vi "Get Data.vi"(8 "error in (no error)":errorcluster, 11 "DAQmx Recorder in":refnum<class "DAQmx Recorder.lvclass">) -> (0 "error out":errorcluster, 2 "Data Result":refnum<class "Acquired Result.lvclass">, 3 "DAQmx Recorder out":refnum<class "DAQmx Recorder.lvclass">)   [LabVIEW 2015, in "DAQmx Recorder.lvclass"]
uses:
  DAQmx Recorder.lvclass
  NHMFL_Core/Libraries/NI-DAQ/DAQmx Digitizer/DAQmx Digitizer.lvclass
  Measure_core/Results/Acquired Result/Acquired Result.lvclass
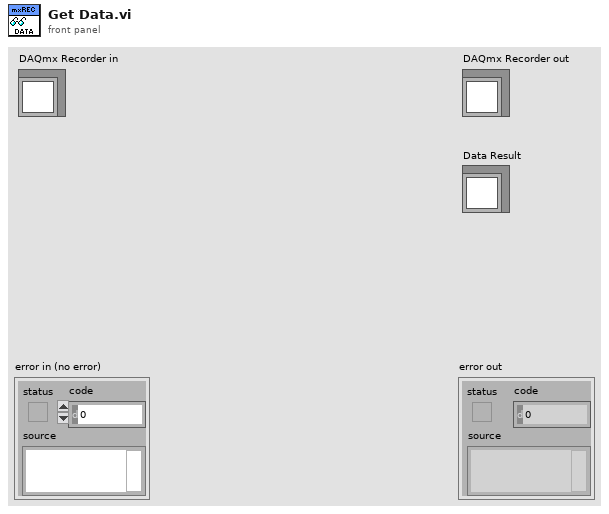
[diagram p1: front panel]
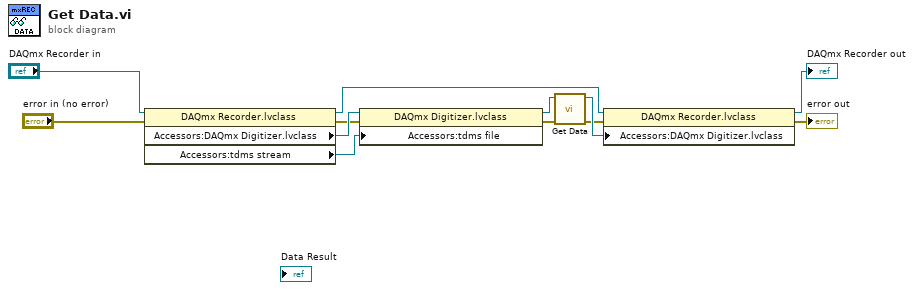
[diagram p0: block diagram]
diagram:
  n1 = property class="DAQmx Recorder.lvclass"(reference="DAQmx Recorder in", error in="error in (no error)") -> (reference out=w5:refnum<class "DAQmx Recorder.lvclass">, error out=w9:errorcluster, "Accessors:DAQmx Digitizer.lvclass"=w10:refnum<class "DAQmx Digitizer.lvclass">, "Accessors:tdms stream"=w11:refnum<k34>)
  n2 = property class="DAQmx Digitizer.lvclass"(reference=w10, error in=w9, "Accessors:tdms file"=w11) -> (reference out=w7:refnum<class "DAQmx Digitizer.lvclass">, error out=w6:errorcluster)
  n3 = call-dynamic "Get Data.vi"("error in (no error)"=w6, "DAQmx Digitizer in"=w7) -> ("error out"=w3:errorcluster, "DAQmx Digitizer out"=w4:refnum<class "DAQmx Digitizer.lvclass">)  [unwired: 8 in]
  n4 = property class="DAQmx Recorder.lvclass"(reference=w5, error in=w3, "Accessors:DAQmx Digitizer.lvclass"=w4) -> (reference out=→"DAQmx Recorder out":refnum<class "DAQmx Recorder.lvclass">, error out=→"error out":errorcluster)
